vi "SimpleView.vi"() -> ()   [LabVIEW 2014]
uses:
  <userlib>/CurtinCode/SimpleViewctrl/SimpleView.xctl
  <userlib>/CurtinCode/Graphctrl/SpectralView.xctl
  <userlib>/CurtinCode/Filexctrl/FilePathControl.xctl
panel:
  in  "FilePathControl":path[](xcontrol)
  out "SpectralView":T1[](xcontrol)
  out "Microphone":T1[](xcontrol)
  out "Spectrum":T1[](xcontrol)
  out "Mag":cluster{i32, dbl, "data":dbl[]}[](graph)=[{0, 3.1467156155762424, "data"=array[8192 elements]}, {0, 3.073180101158845, "data"=array[8192 elements]}, {0, 2.9296875, "data"=array[8192 elements]}, {0, 2.9296875, "data"=array[8192 elements]}, {0, 3.6781609195402303, "data"=array[8192 elements]}]
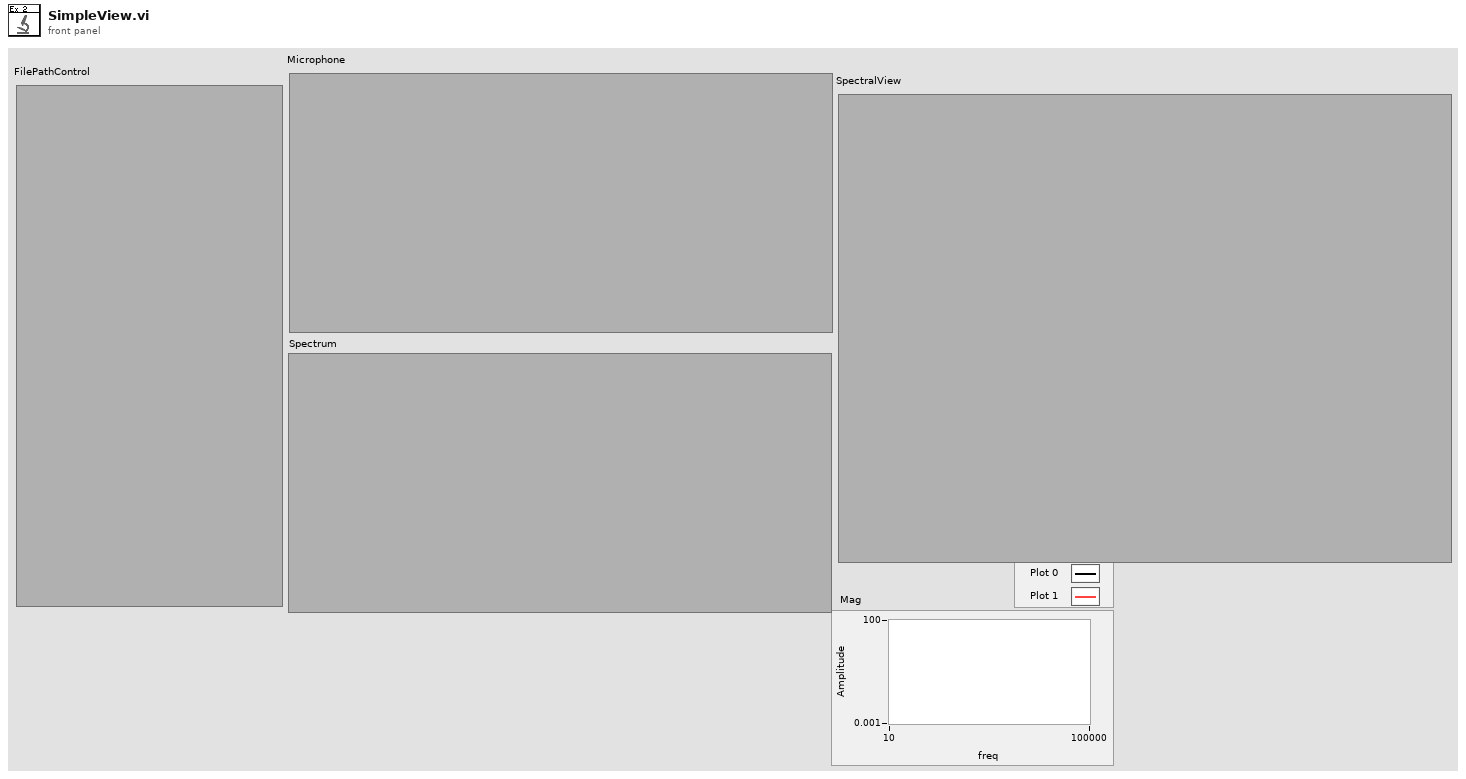
[diagram p1: front panel]
types:
  T1 = typedef "DataControl.ctl" = cluster{"Settings":T2, "Data":cluster{i32, dbl, "data":dbl[]}[], "Plot type":enum16{"Linear", "log"}}
  T2 = typedef "SettingsControl.ctl" = cluster{"Data Path":path, "Time":timestamp, "Sampling Rate (Hz)":u16, "Device":u16, "pre-trigger (sec)":dbl, "length of sample (sec)":dbl, "trigger value (V)":dbl, "Labels":string[], "Cutoffs (sec)":dbl[], "Freq Bands":dbl[]}
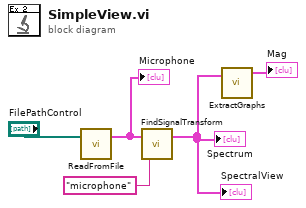
[diagram p0: block diagram]
diagram:
  n1 = call <userlib>:"ReadFromFile.vi"("File paths"="FilePathControl") -> ("Data Sets"=w3:T1[])  [unwired: 1 in, 1 out]
  "Microphone" <- w3
  n2 = call <userlib>:"FindSignalTransform.vi"("Desired data"="microphone" ("Data Set"), "Data Sets In"=w3) -> ("Spectra Out"=w2:T1[])  [unwired: 1 out]
  "Spectrum" <- w2
  "SpectralView" <- w2
  n3 = call <userlib>:"ExtractGraphs.vi"("Spectra Out"=w2) -> ("Mag"=→"Mag":cluster{i32, dbl, "data":dbl[]}[])  [unwired: 3 out]
